vi "Build Instruction List.vi"(7 "Virtual Memory Unit in":refnum<class "Virtual Memory Unit.lvclass">, 8 "error in (no error)":errorcluster, 10 "Starting Address":u16 format="%04x", 11 "Major Frame in":refnum<class "Major Frame.lvclass">) -> (0 "error out":errorcluster, 1 "Instruction List Starting Address":u16, 2 "Next Available Address":u16 format="%04x", 3 "Major Frame out":refnum<class "Major Frame.lvclass">, 4 "Async Pointers":T1 {"HP Async Check Addresses" format="%.0x"; "HP Async Control Addresses" format="%.0x"; "HP Async Data Addresses" format="%.0x"; "LP Async Check Addresses" format="%.0x"; "LP Async Control Addresses" format="%.0x"; "LP Async Data Addresses" format="%.0x"}, 5 "Virtual Memory Unit out":refnum<class "Virtual Memory Unit.lvclass">)   [LabVIEW 2020, in "BCI-1553 API.lvlib" / "Major Frame.lvclass"]
doc: "<DO NOT CALL>\n\nThis method is leveraged by the Bus Controller to properly build the Major Frame sequence.\n\nBuilds the instruction list for a Major Frame."
uses:
  Major Frame.lvclass
  Dependencies/Virtual Memory Unit/Virtual Memory Unit.lvclass
  Major Frame.lvclass/Major Frame.ctl
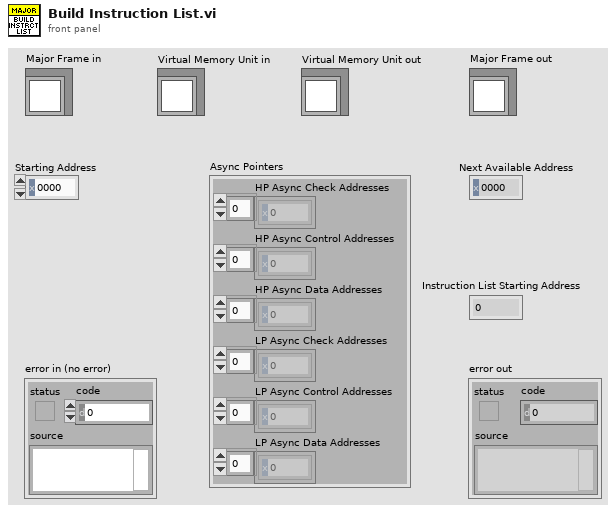
[diagram p1: front panel]
types:
  T1 = cluster{"HP Async Check Addresses":u16[], "HP Async Control Addresses":u16[], "HP Async Data Addresses":u16[], "LP Async Check Addresses":u16[], "LP Async Control Addresses":u16[], "LP Async Data Addresses":u16[]}
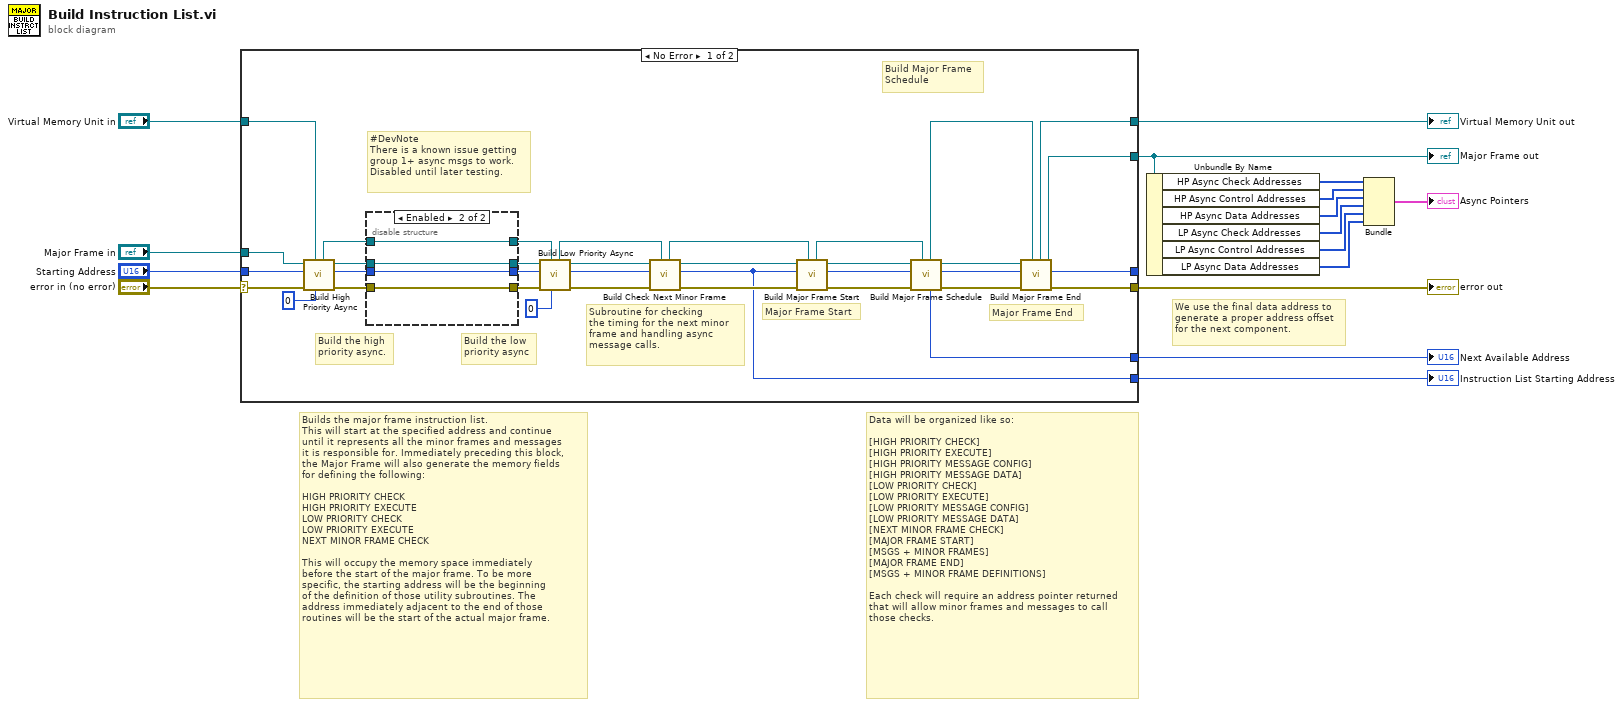
[diagram p0: block diagram]
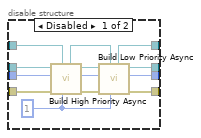
[diagram p2: hidden frame]
diagram:
  # "We use the final data address to\ngenerate a proper address offset\nfor the next component."
  # "Data will be organized like so:\n\n[HIGH PRIORITY CHECK]\n[HIGH PRIORITY EXECUTE]\n[HIGH PRIORITY MESSAGE CONFIG]\n[HIGH PRIORITY MESSAGE DATA]\n[LOW PRIORITY CHECK]\n[LOW PRIORITY EXECUTE]\n[LOW PRIORITY MESSAGE CONFIG]\n[LOW PRIORITY MESSAGE DATA]\n[NEXT MINOR FRAME CHECK]\n[MAJOR FRAME START]\n[MSGS + MINOR FRAMES]\n[MAJOR FRAME END]\n[MSGS + MINOR FRAME DEFINITIONS]\n\nEach check will require an address pointer returned\nthat will allow minor frames and messages to call\nthose checks."
  # "Builds the major frame instruction list.\nThis will start at the specified address and continue\nuntil it represents all the minor frames and messages\nit is responsible for. Immediately preceding this block,\nthe Major Frame will also generate the memory fields\nfor defining the following:\n\nHIGH PRIORITY CHECK\nHIGH PRIORITY EXECUTE\nLOW PRIORITY CHECK\nLOW PRIORITY EXECUTE\nNEXT MINOR FRAME CHECK\n\nThis will occupy the memory space immediately\nbefore the start of the major frame. To be more\nspecific, the starting address will be the beginning\nof the definition of those utility subroutines. The\naddress immediately adjacent to the end of those\nroutines will be the start of the actual major frame."
  n1 = case shown="No Error" "error in (no error)" {
    selector: "error in (no error)" -> [w48 w72]
    tunnel: [w33 w72] -> w15
    tunnel: [w29 w71] -> w10
    tunnel: "Major Frame in" -> [w51 w71]
    tunnel: [w35 w70] -> w13
    tunnel: "Virtual Memory Unit in" -> [w50 w70]
    tunnel: "Starting Address" -> [w49 w69]
    tunnel: [w31 w69] -> _
    tunnel: [w28 _] -> w4
    tunnel: [w27 _] -> w5
    frame No Error {
      # "#DevNote\nThere is a known issue getting\ngroup 1+ async msgs to work.\nDisabled until later testing."
      # "Build the low\npriority async"
      # "Major Frame End"
      # "Build Major Frame\nSchedule"
      # "Major Frame Start"
      # "Subroutine for checking\nthe timing for the next minor\nframe and handling async\nmessage calls."
      # "Build the high\npriority async."
      n2 = call "Build High Priority Async.vi"("Group"=0, "Virtual Memory Unit in"=w50, "error in (no error)"=w48, "Starting Address"=w49, "Major Frame in"=w51) -> ("error out"=w46:errorcluster, "Next Available Address"=w47:u16, "Major Frame out"=w45:refnum<class "Major Frame.lvclass">, "Virtual Memory Unit out"=w44:refnum<class "Virtual Memory Unit.lvclass">)  [unwired: 3 in]
      n3 = disable-structure shown="Enabled" {
        disable-tunnel: w47 -> [w64 w66]
        disable-tunnel: w46 -> [w63 w65]
        disable-tunnel: w45 -> [w62 w67]
        disable-tunnel: w44 -> [w61 w68]
        disable-tunnel: [w60 w65] -> w21
        disable-tunnel: [w59 w66] -> w20
        disable-tunnel: [w58 w67] -> w19
        disable-tunnel: [w57 w68] -> w18
        frame Disabled {
          w52 = 1 ("Group")
          n4 = call "Build High Priority Async.vi"("Group"=w52, "Virtual Memory Unit in"=w61, "error in (no error)"=w63, "Starting Address"=w64, "Major Frame in"=w62) -> ("error out"=w56:errorcluster, "Next Available Address"=w55:u16, "Major Frame out"=w53:refnum<class "Major Frame.lvclass">, "Virtual Memory Unit out"=w54:refnum<class "Virtual Memory Unit.lvclass">)  [unwired: 3 in]
          n5 = call "Build Low Priority Async.vi"("Group"=w52, "Virtual Memory Unit in"=w54, "error in (no error)"=w56, "Starting Address"=w55, "Major Frame in"=w53) -> ("error out"=w60:errorcluster, "Next Available Address"=w59:u16, "Major Frame out"=w58:refnum<class "Major Frame.lvclass">, "Virtual Memory Unit out"=w57:refnum<class "Virtual Memory Unit.lvclass">)  [unwired: 3 in]
        }
        frame Enabled {
        }
      }
      n6 = call "Build Low Priority Async.vi"("Group"=0, "Virtual Memory Unit in"=w18, "error in (no error)"=w21, "Starting Address"=w20, "Major Frame in"=w19) -> ("error out"=w24:errorcluster, "Next Available Address"=w26:u16, "Major Frame out"=w25:refnum<class "Major Frame.lvclass">, "Virtual Memory Unit out"=w22:refnum<class "Virtual Memory Unit.lvclass">)  [unwired: 3 in]
      n7 = call "Build Check Next Minor Frame.vi"("Virtual Memory Unit in"=w22, "error in (no error)"=w24, "Starting Address"=w26, "Major Frame in"=w25) -> ("error out"=w38:errorcluster, "Next Available Address"=w27:u16, "Major Frame out"=w43:refnum<class "Major Frame.lvclass">, "Virtual Memory Unit out"=w41:refnum<class "Virtual Memory Unit.lvclass">)  [unwired: 4 in]
      n8 = call "Build Major Frame Start.vi"("Virtual Memory Unit in"=w41, "error in (no error)"=w38, "Starting Address"=w27, "Major Frame in"=w43) -> ("error out"=w37:errorcluster, "Next Available Address"=w39:u16, "Major Frame out"=w42:refnum<class "Major Frame.lvclass">, "Virtual Memory Unit out"=w40:refnum<class "Virtual Memory Unit.lvclass">)  [unwired: 4 in]
      n9 = call "Build Major Frame Schedule.vi"("Virtual Memory Unit in"=w40, "error in (no error)"=w37, "Starting Address"=w39, "Major Frame in"=w42) -> ("error out"=w34:errorcluster, "Next Available Address"=w32:u16, "Major Frame out"=w30:refnum<class "Major Frame.lvclass">, "Final Data Address"=w28:u16, "Virtual Memory Unit out"=w36:refnum<class "Virtual Memory Unit.lvclass">)  [unwired: 3 in]
      n10 = call "Build Major Frame End.vi"("Virtual Memory Unit in"=w36, "error in (no error)"=w34, "Starting Address"=w32, "Major Frame in"=w30) -> ("error out"=w33:errorcluster, "Next Available Address"=w31:u16, "Major Frame out"=w29:refnum<class "Major Frame.lvclass">, "Virtual Memory Unit out"=w35:refnum<class "Virtual Memory Unit.lvclass">)  [unwired: 4 in]
    }
    frame Error {
    }
  }
  "error out" <- w15
  "Major Frame out" <- w10
  "Virtual Memory Unit out" <- w13
  "Next Available Address" <- w4
  "Instruction List Starting Address" <- w5
  n11 = Unbundle By Name(w10) -> ("HP Async Check Addresses"=w3:u16[], "HP Async Control Addresses"=w9:u16[], "HP Async Data Addresses"=w7:u16[], "LP Async Check Addresses"=w2:u16[], "LP Async Control Addresses"=w6:u16[], "LP Async Data Addresses"=w8:u16[])
  n12 = Bundle("HP Async Check Addresses"=w3, "HP Async Control Addresses"=w9, "HP Async Data Addresses"=w7, "LP Async Check Addresses"=w2, "LP Async Control Addresses"=w6, "LP Async Data Addresses"=w8) -> (→"Async Pointers":T1)  [unwired: 1 in]
